vi "FFT Process.vi"(5 "FFT Parameters":T3={"Direction"=TRUE, "scale_sch"=85.0, "Flush Length"=0} {"scale_sch" format="%.0b"}, 7 "FFT State":cluster{"FFT State":T1, "Set FFT State?":bool}, 8 "Input Valid":bool, 10 "Imag Data In":fxp<+/-,16,1>, 11 "Real Data In":fxp<+/-,16,1>) -> (0 "Output Valid":bool, 1 "Current FFT State":T1, 2 "Imag Data Out":fxp<+/-,16,1> format="%.16g", 3 "Real Data Out":fxp<+/-,16,1> format="%.16g", 4 "FFT Index":fxp<+,9,9>, 6 "FFT Status":T2)   [LabVIEW 2011]
doc: "Note: The first sample of the waveform should begin one cycle after START signal or \"PROCESS STATE\" is enabled"
uses:
  <userlib>/FPGA Library/Code Development/Signal Processing/FFT Block/FFT/Controls/FFT Parameters.ctl
  <userlib>/FPGA Library/Code Development/Signal Processing/FFT Block/FFT/Controls/FFT States.ctl
  <vilib>/rvi/IPIntegrationNode/IPINode_Utilities/niFpgaIPINodeSimCore.vi
  <vilib>/rvi/FXPMathLib/basic elements/FxpDiscreteDelay/XNode/nifxpmath_DiscreteDelay.xnode
  <vilib>/rvi/XilinxIP/XIPIN_XNode/niFpgaXIPIN.xnode
  <userlib>/FPGA Library/Code Development/Signal Processing/FFT Block/FFT/FFT Process/Fast Fourier Transform/FastFourierTransform_F1A05D14459132E02A085DB04D52F246.dll
  <vilib>/rvi/IPIntegrationNode/IPINode_Xnode/niFpgaIPINode.xnode
panel:
  out "rfd":bool
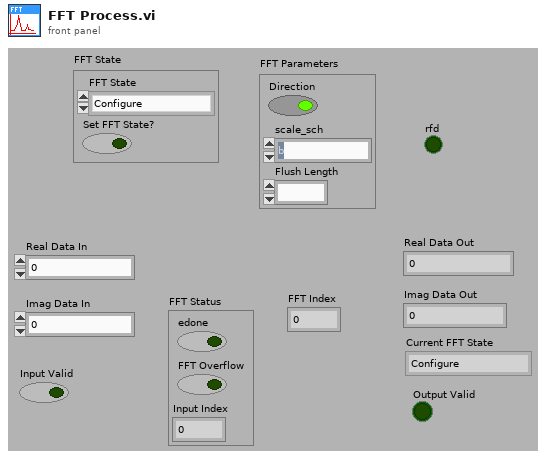
[diagram p1: front panel]
types:
  T1 = typedef "FFT States.ctl" = enum8{"Configure", "Start FFT processing", "Process", "Unload Last FFT", "Reset"}
  T2 = cluster{"edone":bool, "FFT Overflow":bool, "Input Index":fxp<+,9,9>}
  T3 = typedef "FFT Parameters.ctl" = cluster{"Direction":bool, "scale_sch":fxp<+,10,10>, "Flush Length":u16}
  T4 = cluster{"FFT State":enum8{"Configure", "Start FFT processing", "Process", "Unload Last FFT", "Reset"}, "Set FFT State?":bool}
  T5 = cluster{"Direction":bool, "scale_sch":fxp<+,10,10>, "Flush Length":u16}
  T6 = enum8{"Configure", "Start FFT processing", "Process", "Unload Last FFT", "Reset"}
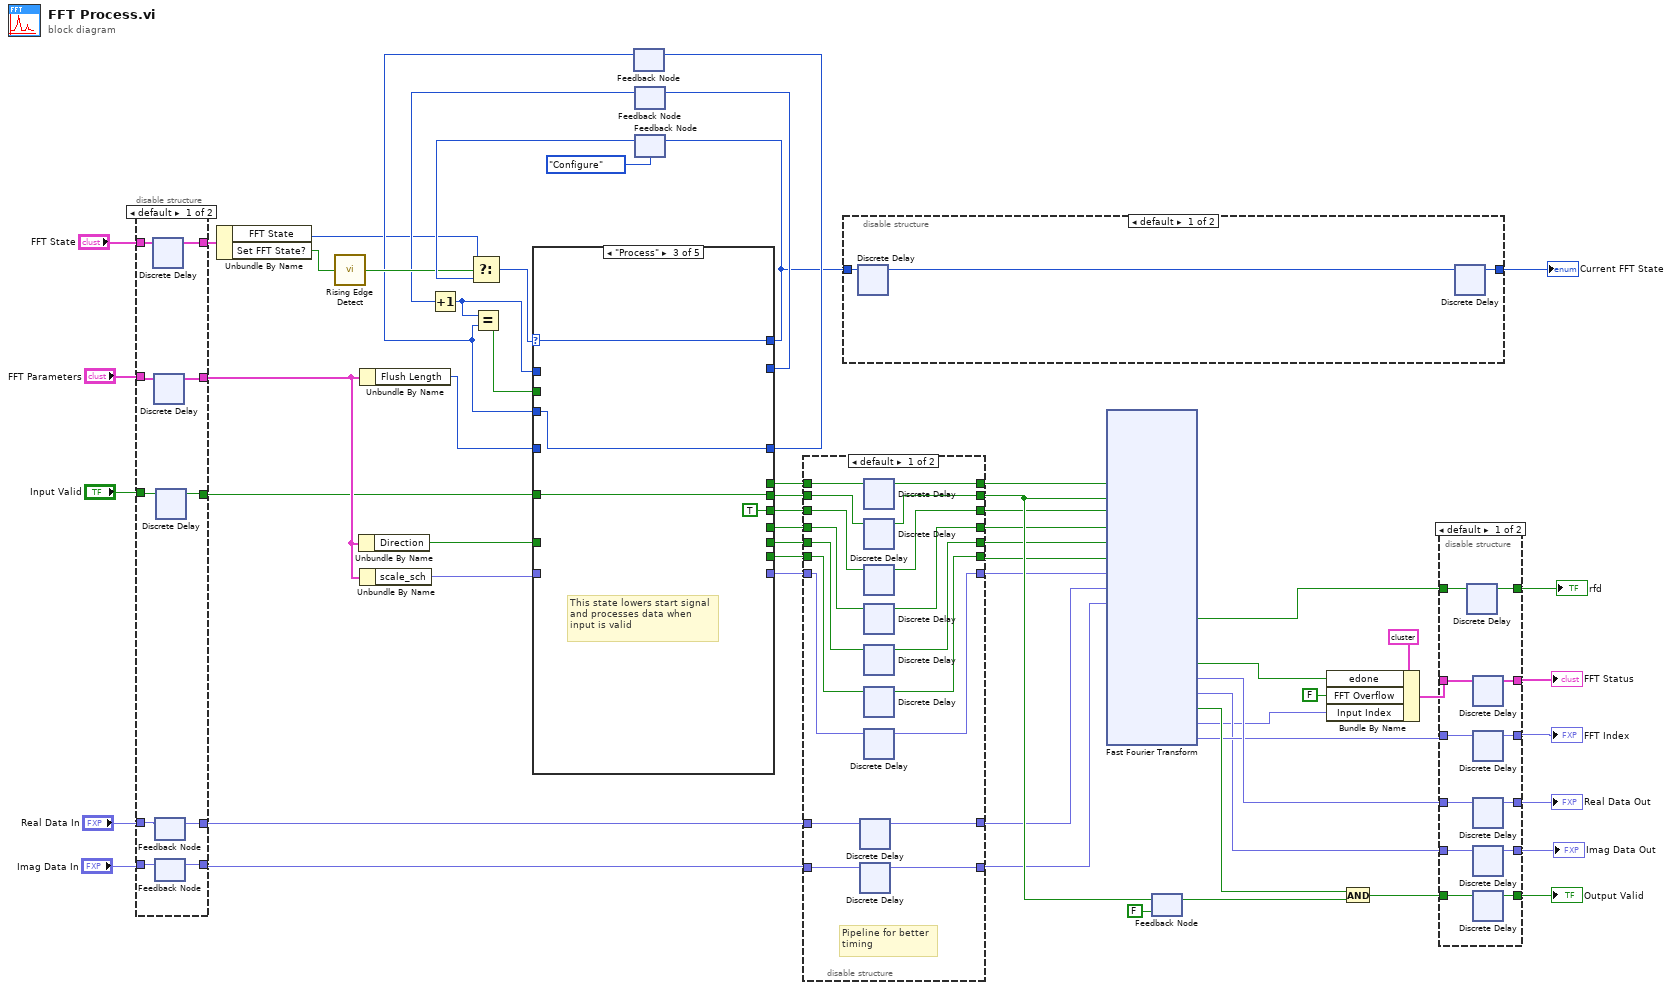
[diagram p0: block diagram]
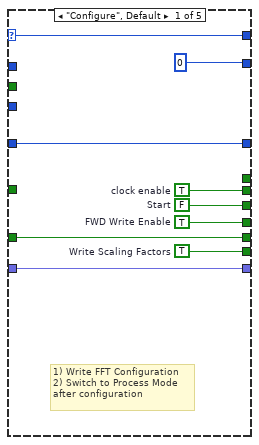
[diagram p6: hidden frame]
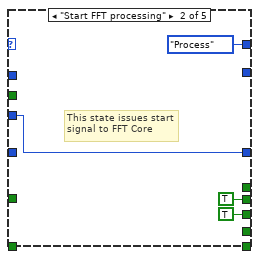
[diagram p7: hidden frame]
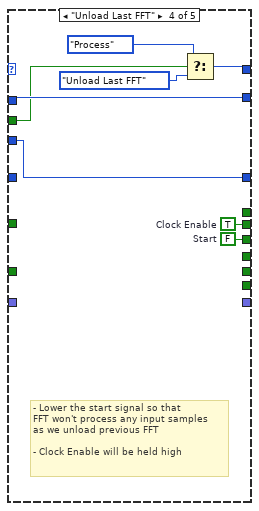
[diagram p8: hidden frame]
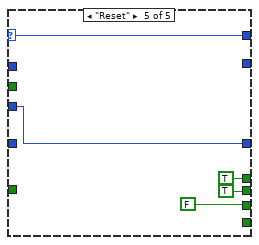
[diagram p9: hidden frame]
diagram:
  n1 = disable-structure shown="default" {
    disable-tunnel: "Input Valid" -> [w64 w75]
    disable-tunnel: "FFT Parameters" -> [w66 w76]
    disable-tunnel: "FFT State" -> [w68 w77]
    disable-tunnel: "Real Data In" -> [w72 w74]
    disable-tunnel: "Imag Data In" -> [w71 w73]
    disable-tunnel: [w67 w77] -> w11
    disable-tunnel: [w65 w76] -> w10
    disable-tunnel: [w63 w75] -> w9
    disable-tunnel: [w70 w74] -> w8
    disable-tunnel: [w69 w73] -> w7
    frame condition #0 (active) {
      n2 = xnode "Discrete Delay"("D"=w68) -> ("Q"=w67:T4)
      n3 = xnode "Discrete Delay"("D"=w66) -> ("Q"=w65:T5)
      n4 = feedback #1() -> (w70:fxp<+/-,16,1>)  [unwired: 1 in]
      n5 = feedback-in #1(w72) -> ()
      n6 = feedback #2() -> (w69:fxp<+/-,16,1>)  [unwired: 1 in]
      n7 = feedback-in #2(w71) -> ()
      n8 = xnode "Discrete Delay"("D"=w64) -> ("Q"=w63:bool)
    }
    frame condition #1 {
    }
  }
  n9 = Unbundle By Name(w11) -> ("FFT State"=w47:T6, "Set FFT State?"=w46:bool)
  n10 = call <userlib>:"Rising Edge Detect.vi"("signal"=w46) -> ("edge detected"=w60:bool)  [unwired: 14 in]
  n11 = Unbundle By Name(w10) -> ("Direction"=w52:bool)
  n12 = Unbundle By Name(w10) -> ("Flush Length"=w53:u16)
  n13 = Unbundle By Name(w10) -> ("scale_sch"=w50:fxp<+,10,10>)
  n14 = feedback #3() -> (w54:u16)  [unwired: 1 in]
  n15 = feedback #4() -> (w59:u16)  [unwired: 1 in]
  n16 = Increment(x=w59) -> (x+1=w56:u16)
  n17 = Equal?(x=w56, y=w54) -> (x = y?=w55:bool)
  n18 = feedback #5(FFT_States."Configure" ("FFT State")) -> (w61:T1)
  n19 = Select(t=w47, s=w60, f=w61) -> (s? t:f=w44:T1)
  n20 = case shown="\"Process\"" w44 {
    selector: w44 -> [w86 _ w94 _ w106]
    tunnel: w9 -> [_ _ w91 _ _]
    tunnel: [w86 FFT_States."Process" ("FFT State") w94 w98 w106] -> w36
    tunnel: w50 -> [w81 _ _ _ _]
    tunnel: w52 -> [w82 _ _ _ _]
    tunnel: [w85 TRUE ("Clock Enable") w91 w102 TRUE ("Clock Enable")] -> w24
    tunnel: [w84 TRUE ("Start") TRUE ("Start") w101 FALSE ("Start")] -> w29
    tunnel: [w83 _ _ _ _] -> w30
    tunnel: [w82 _ _ _ _] -> w28
    tunnel: [w81 _ _ _ _] -> w32
    tunnel: [w80 _ _ _ _] -> w31
    tunnel: [_ _ _ _ TRUE] -> w33
    tunnel: [u16 0 _ _ w100 _] -> w58
    tunnel: w56 -> [_ _ _ w100 _]
    tunnel: w53 -> [w78 _ _ _ _]
    tunnel: [w78 w89 w92 w97 w107] -> w57
    tunnel: w54 -> [_ w89 w92 w97 w107]
    tunnel: w55 -> [_ _ _ w99 _]
    frame "Configure", Default {
      w80 = TRUE  # Write Scaling Factors
      w83 = TRUE  # FWD Write Enable
      w84 = FALSE  # Start
      w85 = TRUE  # clock enable
      # "1) Write FFT Configuration\n2) Switch to Process Mode\nafter configuration"
    }
    frame "Start FFT processing" {
      # "This state issues start\nsignal to FFT Core"
    }
    frame "Process" {
      # "This state lowers start signal\nand processes data when\ninput is valid"
    }
    frame "Unload Last FFT" {
      w101 = FALSE  # Start
      w102 = TRUE  # Clock Enable
      # "- Lower the start signal so that\nFFT won't process any input samples\nas we unload previous FFT\n\n- Clock Enable will be held high"
      n21 = Select(t=FFT_States."Process" ("FFT State"), s=w99, f=FFT_States."Unload Last FFT" ("FFT State")) -> (s? t:f=w98:T1)
    }
    frame "Reset" {
    }
  }
  n22 = feedback-in #3(w57) -> ()
  n23 = feedback-in #4(w58) -> ()
  n24 = feedback-in #5(w36) -> ()
  n25 = disable-structure shown="default" {
    disable-tunnel: w33 -> [w125 w134]
    disable-tunnel: w32 -> [w124 w128]
    disable-tunnel: w31 -> [w123 w129]
    disable-tunnel: w30 -> [w122 w131]
    disable-tunnel: w29 -> [w121 w132]
    disable-tunnel: w28 -> [w120 w130]
    disable-tunnel: w24 -> [w119 w133]
    disable-tunnel: [w118 w134] -> w20
    disable-tunnel: [w117 w133] -> w19
    disable-tunnel: [w116 w132] -> w18
    disable-tunnel: [w115 w131] -> w17
    disable-tunnel: [w114 w130] -> w16
    disable-tunnel: [w113 w129] -> w3
    disable-tunnel: [w112 w128] -> w2
    disable-tunnel: w8 -> [w111 w127]
    disable-tunnel: [w110 w127] -> w14
    disable-tunnel: [w109 w126] -> w13
    disable-tunnel: w7 -> [w108 w126]
    frame condition #0 (active) {
      # "Pipeline for better\ntiming"
      n26 = xnode "Discrete Delay"("D"=w111) -> ("Q"=w110:fxp<+/-,16,1>)
      n27 = xnode "Discrete Delay"("D"=w108) -> ("Q"=w109:fxp<+/-,16,1>)
      n28 = xnode "Discrete Delay"("D"=w125) -> ("Q"=w118:bool)
      n29 = xnode "Discrete Delay"("D"=w119) -> ("Q"=w117:bool)
      n30 = xnode "Discrete Delay"("D"=w121) -> ("Q"=w116:bool)
      n31 = xnode "Discrete Delay"("D"=w122) -> ("Q"=w115:bool)
      n32 = xnode "Discrete Delay"("D"=w120) -> ("Q"=w114:bool)
      n33 = xnode "Discrete Delay"("D"=w123) -> ("Q"=w113:bool)
      n34 = xnode "Discrete Delay"("D"=w124) -> ("Q"=w112:fxp<+,10,10>)
    }
    frame condition #1 {
    }
  }
  n35 = disable-structure shown="default" {
    disable-tunnel: [w137 w138] -> w25
    disable-tunnel: w36 -> [w136 w138]
    frame condition #0 (active) {
      n36 = xnode "Discrete Delay"("D"=w136) -> ("Q"=w135:T6)
      n37 = xnode "Discrete Delay"("D"=w135) -> ("Q"=w137:T6)
    }
    frame condition #1 {
    }
  }
  "Current FFT State" <- w25
  n38 = xnode ("Fast Fourier Transform")("sclr"=w20, "ce"=w19, "start"=w18, "fwd_inv_we"=w17, "fwd_inv"=w16, "scale_sch_we"=w3, "scale_sch"=w2, "xn_re"=w14, "xn_im"=w13) -> ("rfd"=w5:bool, "edone"=w43:bool, "xk_re"=w23:fxp<+/-,16,1>, "xk_im"=w21:fxp<+/-,16,1>, "dv"=w35:bool, "xn_index"=w1:fxp<+,10,10>, "xk_index"=w22:fxp<+,10,10>)  [unwired: 2 out]
  n39 = feedback-in #6(w19) -> ()
  n40 = feedback #6(FALSE ("Clock Enable")) -> (w27:bool)
  n41 = Bundle By Name(cluster=T2 {"edone"=FALSE, "FFT Overflow"=FALSE, "Input Index"=0.0} ("Cluster"), "edone"=w43, "FFT Overflow"=FALSE, "Input Index"=w1) -> (w42:T2)
  n42 = And(x=w35, y=w27) -> (x .and. y?=w34:bool)
  n43 = disable-structure shown="default" {
    disable-tunnel: w21 -> [w150 w153]
    disable-tunnel: w23 -> [w149 w154]
    disable-tunnel: w42 -> [w148 w156]
    disable-tunnel: w22 -> [w147 w155]
    disable-tunnel: [w146 w156] -> w41
    disable-tunnel: [w145 w155] -> w40
    disable-tunnel: [w144 w154] -> w39
    disable-tunnel: [w143 w153] -> w38
    disable-tunnel: [w142 w152] -> w37
    disable-tunnel: w34 -> [w141 w152]
    disable-tunnel: w5 -> [w140 w151]
    disable-tunnel: [w139 w151] -> w4
    frame condition #0 (active) {
      n44 = xnode "Discrete Delay"("D"=w140) -> ("Q"=w139:bool)
      n45 = xnode "Discrete Delay"("D"=w148) -> ("Q"=w146:T2)
      n46 = xnode "Discrete Delay"("D"=w147) -> ("Q"=w145:fxp<+,10,10>)
      n47 = xnode "Discrete Delay"("D"=w149) -> ("Q"=w144:fxp<+/-,16,1>)
      n48 = xnode "Discrete Delay"("D"=w150) -> ("Q"=w143:fxp<+/-,16,1>)
      n49 = xnode "Discrete Delay"("D"=w141) -> ("Q"=w142:bool)
    }
    frame condition #1 {
    }
  }
  "Output Valid" <- w37
  "Imag Data Out" <- w38
  "Real Data Out" <- w39
  "FFT Status" <- w41
  "FFT Index" <- w40
  "rfd" <- w4
